vi "Read MsgPackMessage.vi"(8 "error in (no error)":errorcluster, 11 "IMsgPackMessageHandler in":refnum<class "IMsgPackMessageHandler.lvclass">) -> (0 "error out":errorcluster, 2 "wamplv.lvlib:MsgPackMessage.lvclass":refnum<class "MsgPackMessage.lvclass">, 3 "IMsgPackMessageHandler out":refnum<class "IMsgPackMessageHandler.lvclass">)   [LabVIEW 2020, in "wamplv.lvlib" / "IMsgPackMessageHandler.lvclass"]
uses:
  IMsgPackMessageHandler.lvclass
  IMsgPackMessageHandler.lvclass/IMsgPackMessageHandler.ctl
  SerialisedMessages/MsgPackMessage/MsgPackMessage.lvclass
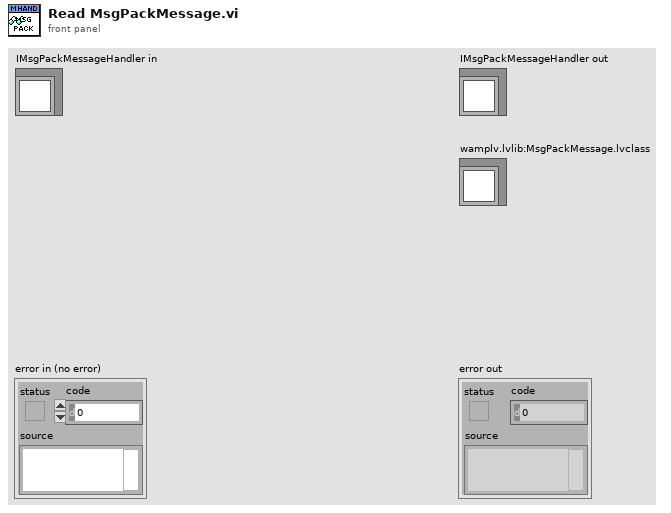
[diagram p1: front panel]
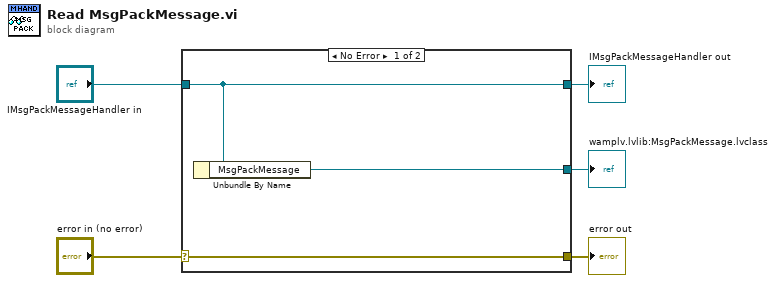
[diagram p0: block diagram]
diagram:
  n1 = case shown="No Error" "error in (no error)" {
    selector: "error in (no error)" -> [w8 w9]
    tunnel: [w8 w9] -> w4
    tunnel: [w7 w10] -> w2
    tunnel: "IMsgPackMessageHandler in" -> [w7 w10]
    tunnel: [w6 _] -> w1
    frame No Error {
      n2 = Unbundle By Name(w7) -> ("MsgPackMessage"=w6:refnum<class "MsgPackMessage.lvclass">)
    }
    frame Error {
    }
  }
  "error out" <- w4
  "IMsgPackMessageHandler out" <- w2
  "wamplv.lvlib:MsgPackMessage.lvclass" <- w1
